vi "Write Lock-in driver.vi"(8 "error in (no error)":errorcluster, 10 "Lock-in Driver.lvclass":refnum<class "Lock-in Driver.lvclass">, 11 "Lock-in in":refnum<class "Lock-in.lvclass">) -> (0 "error out":errorcluster, 3 "Lock-in out":refnum<class "Lock-in.lvclass">)   [LabVIEW 2019, in "Lock-in.lvclass"]
uses:
  Lock-in.lvclass
  C:/GitHub/LabActor/Instrument Actor/Instrument Actor.lvclass
  NHMFL_Core/Libraries/Instruments/Instrument Driver/Lock-in Driver/Lock-in Driver.lvclass
  C:/GitHub/NHMFL_Core/Libraries/Instruments/Instrument Driver/Instrument Driver.lvclass
  Instrument Actor/Instrument Actor.lvclass/Instrument Actor.ctl
  Instrument Actor/Write Instrument driver.vi
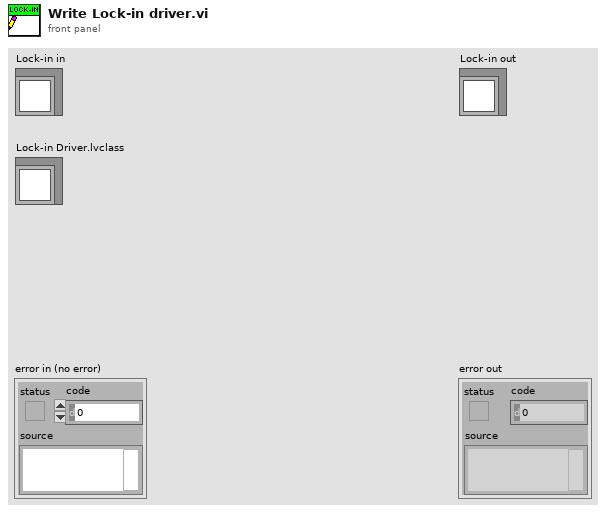
[diagram p1: front panel]
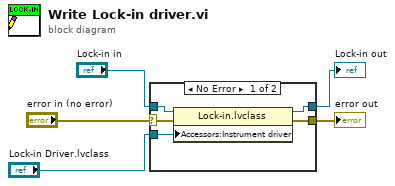
[diagram p0: block diagram]
diagram:
  n1 = case shown="No Error" "error in (no error)" {
    selector: "error in (no error)" -> [w7 w11]
    tunnel: [w6 w11] -> w4
    tunnel: [w9 w12] -> w2
    tunnel: "Lock-in in" -> [w10 w12]
    tunnel: "Lock-in Driver.lvclass" -> [w8 _]
    frame No Error {
      n2 = property class="Lock-in.lvclass"(reference=w10, error in=w7, "Accessors:Instrument driver"=w8) -> (reference out=w9:refnum<class "Lock-in.lvclass">, error out=w6:errorcluster)
    }
    frame Error {
    }
  }
  "error out" <- w4
  "Lock-in out" <- w2
